vi "path_data.vi"(10 "path in":dbl[][](array[numeric]), 11 "increment":dbl) -> (3 "path logical":dbl[](array[numeric]))   [LabVIEW 2015]
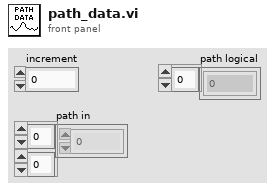
[diagram p1: front panel]
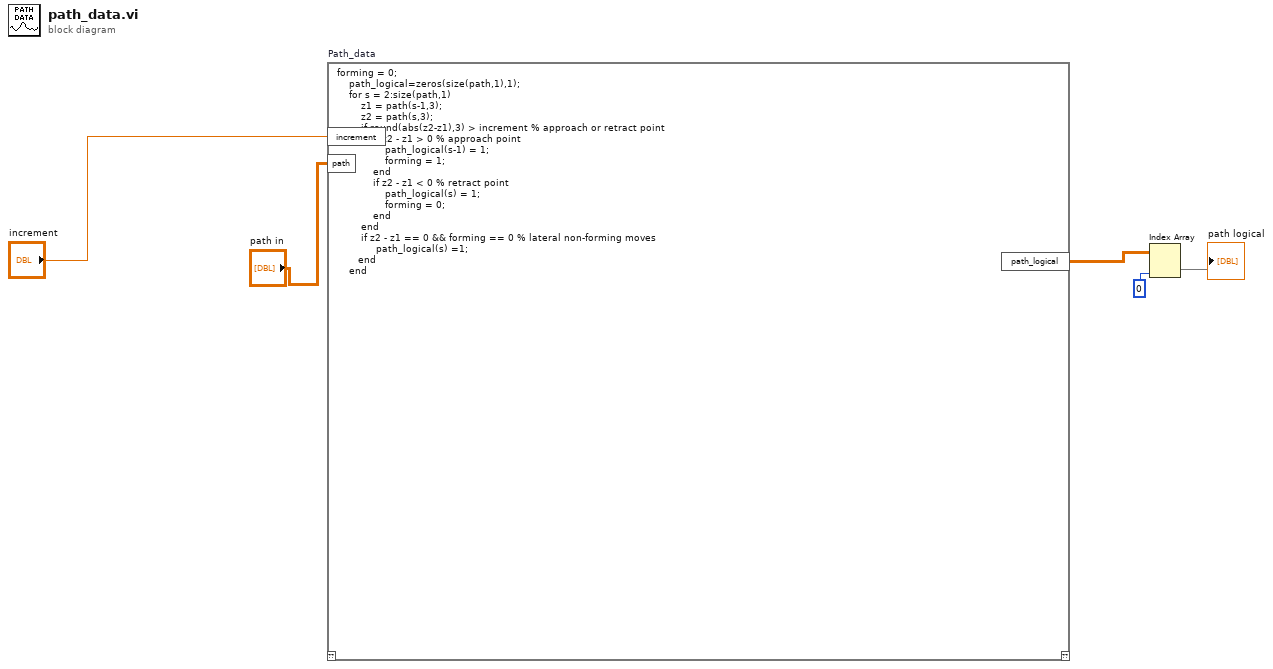
[diagram p0: block diagram]
diagram:
  n1 = script code="forming = 0;\n    path_logical=zeros(size(path,1),1);\n    for s = 2:size(path,1)\n        z1 = path(s-1,3);\n        z2 = path(s,3);\n        if round(abs(z2-z1),3) > increment % approach or retract point\n            if z2 - z1 > 0 % approach point\n                path_logical(s-1) = 1;\n                forming = 1;\n            end\n            if z2 - z1 < 0 % retract point\n                path_logical(s) = 1;\n                forming = 0;\n            end\n        end\n        if z2 - z1 == 0 && forming == 0 % lateral non-forming moves\n             path_logical(s) =1;\n       end\n    end" "Path_data"("increment"="increment", "path"="path in") -> ("path_logical"=w3:dbl[][])  [unwired: 1 in, 1 out]
  n2 = Index Array(array=w3, index (col)=0 ("disabled index (col)")) -> (element=→"path logical":dbl[])  [unwired: 1 in]
